vi "Cockpit UDP Test.vi"() -> ()   [LabVIEW 2010]
panel:
  out "Waveform Chart 5":sgl(graph)
  out "Waveform Chart 4":sgl(graph)
  out "Waveform Chart 3":sgl(graph)
  out "Waveform Chart 2":sgl(graph)
  out "Waveform Chart 1":sgl(graph)
  in  "UDP write":dbl[](array[numeric])
  in  "stop":bool
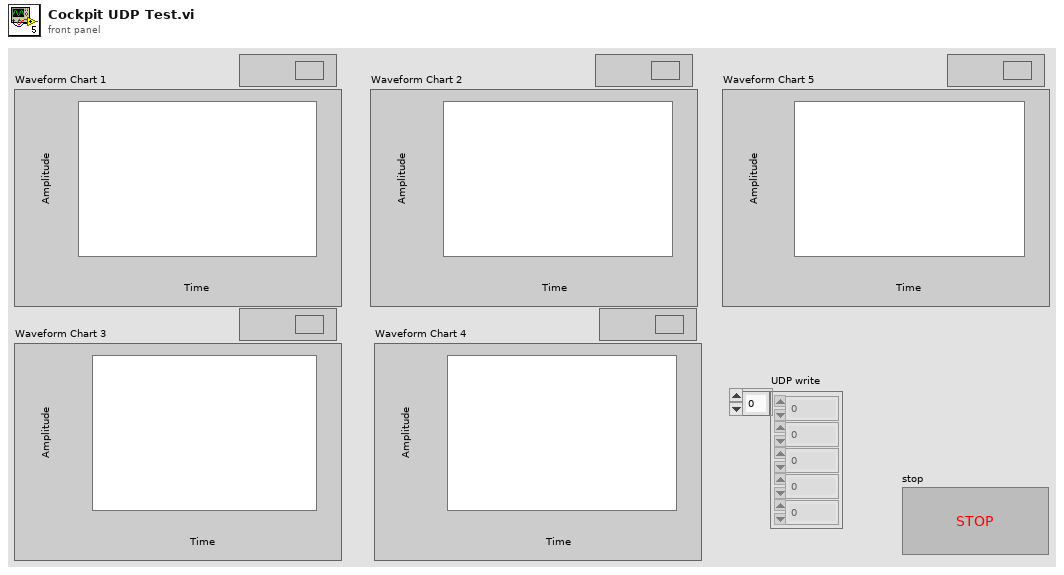
[diagram p1: front panel]
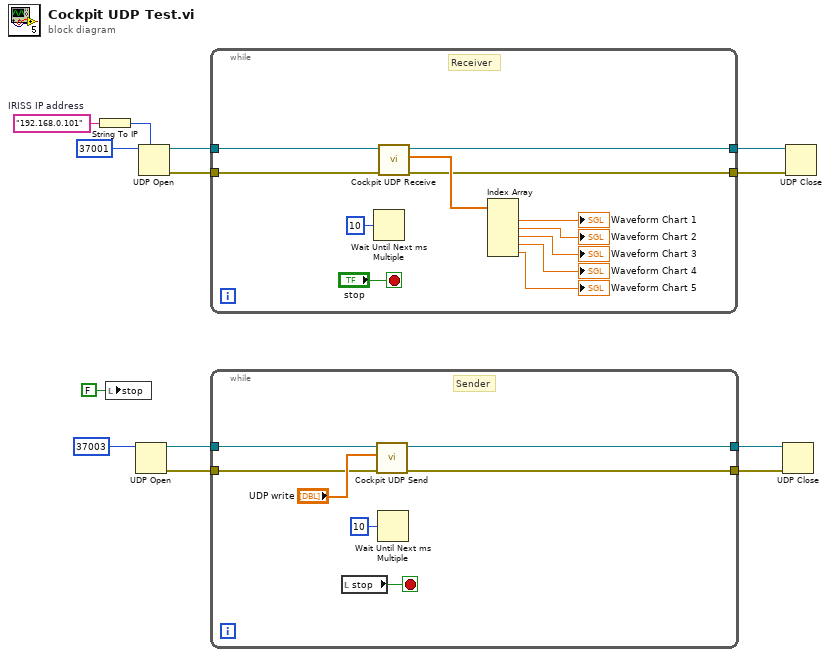
[diagram p0: block diagram]
diagram:
  w6 = "192.168.0.101"  # IRISS IP address
  n1 = String To IP(1:w6) -> (0:w7:u32)
  n2 = local write "stop"(FALSE ("stop")) -> ()
  n3 = UDP Open(11:u16 37003 ("port")) -> (port=w12:refnum<k16>, 0:w11:errorcluster)  [unwired: 4 in, 1 out]
  n4 = UDP Open(7:w7, 11:u16 37001 ("port")) -> (port=w4:refnum<k16>, 0:w3:errorcluster)  [unwired: 3 in, 1 out]
  n5 = while {
    tunnel: w4 -> [w22]
    tunnel: w3 -> [w21]
    tunnel: [w15] -> w2
    tunnel: [w14] -> w1
    stop <- "stop" stop-if-true
    # "Receiver"
    n6 = Wait Until Next ms Multiple(millisecond multiple=u32 10) -> ()  [unwired: 1 out]
    n7 = call "Cockpit UDP Receive.vi"("error in"=w21, "connection ID"=w22) -> ("error out"=w14:errorcluster, "read UDP array"=w24:sgl[], "connection ID out"=w15:refnum<k16>)  [unwired: 7 in]
    n8 = Index Array(array=w24) -> (element #1=→"Waveform Chart 1":sgl, element #2=→"Waveform Chart 2":sgl, element #3=→"Waveform Chart 3":sgl, element #4=→"Waveform Chart 4":sgl, element #5=→"Waveform Chart 5":sgl)  [unwired: 5 in]
  }
  n9 = while {
    tunnel: w12 -> [w29]
    tunnel: w11 -> [w28]
    tunnel: [w27] -> w10
    tunnel: [w26] -> w9
    stop <- w30 stop-if-true
    # "Sender"
    n10 = local read "stop"() -> (w30:bool)
    n11 = call "Cockpit UDP Send.vi"("error in"=w28, "write UDP array"="UDP write", "connection ID"=w29) -> ("error out"=w26:errorcluster, "connection ID out"=w27:refnum<k16>)  [unwired: 7 in]
    n12 = Wait Until Next ms Multiple(millisecond multiple=u32 10) -> ()  [unwired: 1 out]
  }
  n13 = UDP Close(connection ID=w10, 8:w9) -> ()  [unwired: 2 out]
  n14 = UDP Close(connection ID=w2, 8:w1) -> ()  [unwired: 2 out]
